vi "Layout - ISO 8601 timestamp.vi"(8 "error in (no error)":errorcluster) -> (0 "error out":errorcluster)   [LabVIEW 2026, in "Tests.lvlib"]
doc: "Unit test (Caraya). Verifies FormatTimeString renders ISO 8601 with millisecond precision: a UTC instant formats as YYYY-MM-DDThh:mm:ss.mmmZ, the fractional field is correct, and a local-frame instant renders its wall-clock (offset not asserted, as it is machine-dependent). Inputs are built with Date/Time To Seconds so the instant is deterministic. Pure, no fixtures.\n\nImplements LMBR-T-004 -> SRS-011. Assert-level IDs: Test-ID-Assert-Checklist.md."
uses:
  Tests.lvlib
  <vilib>/Utility/miscctls.llb/LVDateTimeRec.ctl
  <vilib>/addons/_JKI Toolkits/Caraya/classes/Assert/Assert Equal Value_Variant.vi
  <vilib>/addons/_JKI Toolkits/Caraya/classes/Test/Test.lvclass
  <vilib>/addons/_JKI Toolkits/Caraya/classes/Assert/Assert.lvclass
  src/Lumberjack.lvlib
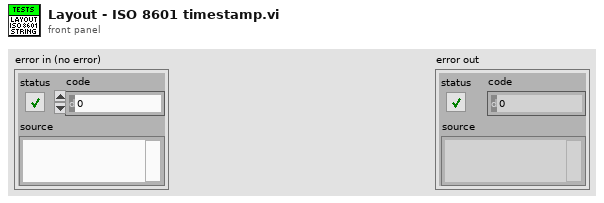
[diagram p1: front panel]
types:
  T1 = typedef "LVDateTimeRec.ctl" = cluster{"fractional second":dbl, "second":i32, "minute":i32, "hour":i32, "day of month":i32, "month":i32, "year":i32, "day of week":i32, "day of year":i32, "DST":i32}
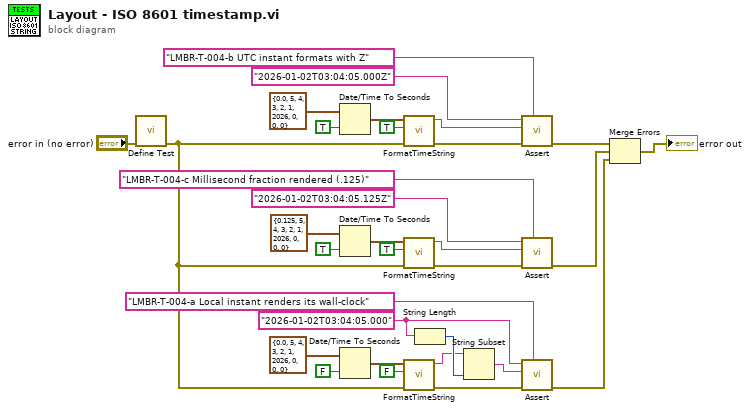
[diagram p0: block diagram]
diagram:
  w4 = "2026-01-02T03:04:05.000" ("raw")
  n1 = call <vilib>:"Define Test.vi"("error in (no error)"="error in (no error)") -> ("error out"=w31:errorcluster)  [unwired: 9 in, 1 out]
  n2 = Date/Time To Seconds(1:TRUE ("is UTC (F)"), 2:T1 {"fractional second"=0.0, "second"=5, "minute"=4, "hour"=3, "day of month"=2, "month"=1, "year"=2026, "day of week"=0, "day of year"=0, "DST"=0} ("date time rec")) -> (0:w11:timestamp)
  n3 = Date/Time To Seconds(1:TRUE ("is UTC (F)"), 2:T1 {"fractional second"=0.125, "second"=5, "minute"=4, "hour"=3, "day of month"=2, "month"=1, "year"=2026, "day of week"=0, "day of year"=0, "DST"=0} ("date time rec")) -> (0:w8:timestamp)
  n4 = Date/Time To Seconds(1:FALSE ("is UTC (F)"), 2:T1 {"fractional second"=0.0, "second"=5, "minute"=4, "hour"=3, "day of month"=2, "month"=1, "year"=2026, "day of week"=0, "day of year"=0, "DST"=0} ("date time rec")) -> (0:w5:timestamp)
  n5 = call "FormatTimeString.vi"("error in (no error)"=w31, "useUTC"=TRUE, "timestamp"=w11) -> ("error out"=w29:errorcluster, "timeString"=w28:string)  [unwired: 7 in]
  n6 = call "FormatTimeString.vi"("error in (no error)"=w31, "useUTC"=TRUE, "timestamp"=w8) -> ("error out"=w24:errorcluster, "timeString"=w23:string)  [unwired: 7 in]
  n7 = call "FormatTimeString.vi"("error in (no error)"=w31, "useUTC"=FALSE, "timestamp"=w5) -> ("error out"=w20:errorcluster, "timeString"=w2:string)  [unwired: 7 in]
  n8 = String Length(string=w4) -> (length=w3:i32)
  n9 = String Subset(string=w2, length (rest)=w3) -> (substring=w1:string)  [unwired: 1 in]
  n10 = call-poly <vilib>:"Assert.vi"("Label"="LMBR-T-004-b UTC instant formats with Z", "error in (no error)"=w29, "Actual"=w28, "Expected"="2026-01-02T03:04:05.000Z" ("raw")) -> ("error out"=w26:errorcluster)  [unwired: 6 in, 1 out]
  n11 = call-poly <vilib>:"Assert.vi"("Label"="LMBR-T-004-c Millisecond fraction rendered (.125)", "error in (no error)"=w24, "Actual"=w23, "Expected"="2026-01-02T03:04:05.125Z" ("raw")) -> ("error out"=w18:errorcluster)  [unwired: 6 in, 1 out]
  n12 = call-poly <vilib>:"Assert.vi"("Label"="LMBR-T-004-a Local instant renders its wall-clock", "error in (no error)"=w20, "Actual"=w1, "Expected"=w4) -> ("error out"=w17:errorcluster)  [unwired: 6 in, 1 out]
  n13 = Merge Errors(w26, w18, w17) -> (→"error out":errorcluster)
